vi "MoveHatchIntake-C.vi"(11 "Params":string[][](array[string])) -> ()   [LabVIEW 2018]
uses:
  Framework/Robot Global Data.vi
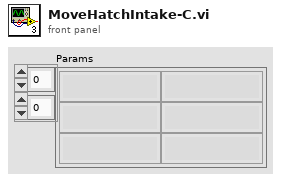
[diagram p1: front panel]
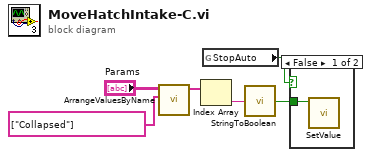
[diagram p0: block diagram]
diagram:
  n1 = call "ArrangeValuesByName.vi"("Names"=string[] ["Collapsed"], "Names/Values in"="Params") -> ("Values Out"=w2:string[])  [unwired: 9 in]
  n2 = Index Array(array=w2) -> (element=w1:string)  [unwired: 1 in]
  n3 = global read "Robot Global Data.vi" "StopAuto"() -> (w5:bool)
  n4 = call "StringToBoolean.vi"("String"=w1) -> ("Output"=w6:bool)
  n5 = case shown="False" w5 {
    tunnel: w6 -> [w7 _]
    frame False {
      n6 = call "SetValue.vi"("Value"=w7) -> ()  [unwired: 10 in, 1 out]
    }
    frame True {
    }
  }
